vi "GetDynamicModules.vi"(8 "error in (no error)":errorcluster, 11 "modules":T1[](array[typedef])) -> (0 "error out":errorcluster, 2 "number of dynamic modules":i32, 3 "all dynamic modules":string[](array[string]))   [LabVIEW 2017, in "CmsFpgaBitfileManager.lvlib"]
uses:
  <vilib>/addons/InsightCM/Devices/Shared/Cms/CmsFpgaBitfileManager/CmsFpgaBitfileManager.lvlib
  <vilib>/addons/cRIODetectHW/control/cRIO Product Info.ctl
  <vilib>/addons/cRIODetectHW/cRIODetectHW.lvlib
panel:
  out "all scan modules":string[](array[string])
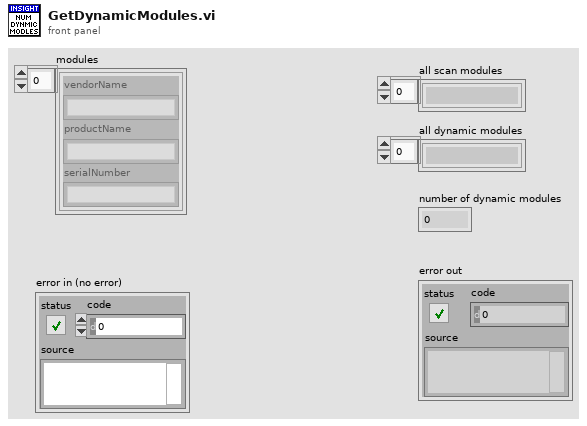
[diagram p1: front panel]
types:
  T1 = typedef "cRIODetectHW.lvlib/cRIO Product Info.ctl" = cluster{"vendorName":string, "productName":string, "serialNumber":string}
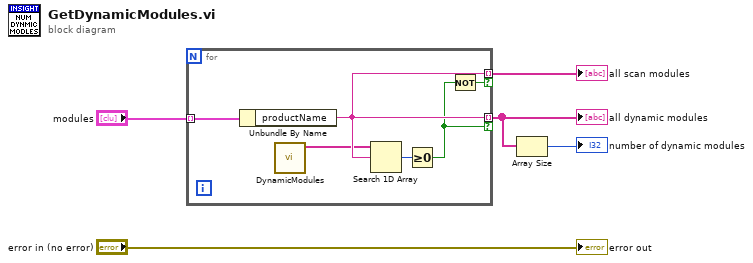
[diagram p0: block diagram]
diagram:
  n1 = for {
    tunnel: "modules" -> [w10] mode=indexing
    tunnel: [w9] -> w3 mode=indexing if=w8
    tunnel: [w9] -> w1 mode=indexing if=w7
    n2 = Unbundle By Name(w10) -> ("productName"=w9:string)
    n3 = call <vilib>:"DynamicModules.vi"() -> ("dynamic modules"=w6:string[])  [unwired: 11 in]
    n4 = Search 1D Array(1D array=w6, element=w9) -> (index of element=w11:i32)  [unwired: 1 in]
    n5 = Greater Or Equal To 0?(x=w11) -> (x >= 0?=w8:bool)
    n6 = Not(x=w8) -> (.not. x?=w7:bool)
  }
  "all dynamic modules" <- w3
  "all scan modules" <- w1
  n7 = Array Size(array=w3) -> (size(s)=→"number of dynamic modules":i32)
  "error out" <- "error in (no error)"
